vi "Shoot preset find corresponding RPM.vi"(1 "Shooter Preset speeds (RPM)":T1=enum."Target Zone") -> (0 "Shooter Speed (RPM)":dbl)   [LabVIEW 2019]
uses:
  Shooter Preset speeds Type Def.ctl
  <vilib>/gmath/NI_Gmath.lvlib
panel:
  in  "Shooter Values":dbl[][](array[numeric])=[[0.0, 0.0], [1.0, 500.0], [2.0, 1000.0], [3.0, 2000.0], [4.0, 3000.0]]
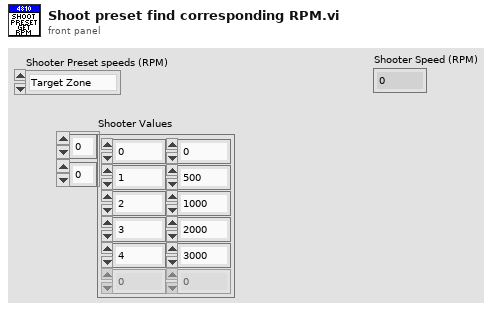
[diagram p1: front panel]
types:
  T1 = typedef "Shooter Preset speeds Type Def.ctl" = enum16{"Not Applicable", "Target Zone", "Initiation Line", "Close end of Trench Run", "Control Panel"}
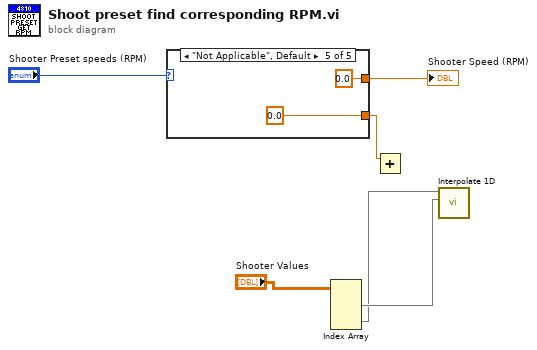
[diagram p0: block diagram]
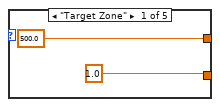
[diagram p2: hidden frame]
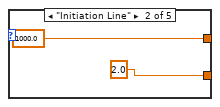
[diagram p3: hidden frame]
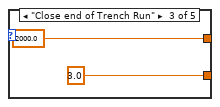
[diagram p4: hidden frame]
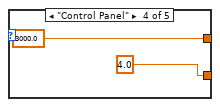
[diagram p5: hidden frame]
diagram:
  n1 = case shown="\"Not Applicable\", Default" "Shooter Preset speeds (RPM)" {
    tunnel: [500.0 ("Shooter Speed (RPM)") 1000.0 ("Shooter Speed (RPM)") 2000.0 ("Shooter Speed (RPM)") 3000.0 ("Shooter Speed (RPM)") 0.0 ("Shooter Speed (RPM)")] -> w5
    tunnel: [1.0 2.0 3.0 4.0 0.0] -> w1
    frame "Target Zone" {
    }
    frame "Initiation Line" {
    }
    frame "Close end of Trench Run" {
    }
    frame "Control Panel" {
    }
    frame "Not Applicable", Default {
    }
  }
  "Shooter Speed (RPM)" <- w5
  n2 = Index Array(array="Shooter Values") -> (element #1=w3:dbl[], element #2=w2:dbl[])  [unwired: 4 in]
  n3 = Add(x=w1) -> ()  [unwired: 1 in, 1 out]
  n4 = call <vilib>:"Interpolate 1D.vi"("X"=w3, "Y"=w2) -> ()  [unwired: 7 in, 3 out]
